vi "SRU2（DBL）.vi"(6 "复位":bool, 7 "启用（T）":bool=TRUE, 9 "初始值":dbl, 10 "Xi":dbl) -> (1 "Xi-1":dbl format="%.2f", 2 "Xi-2":dbl format="%.2f")   [LabVIEW 2012]
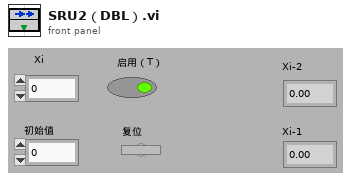
[diagram p1: front panel]
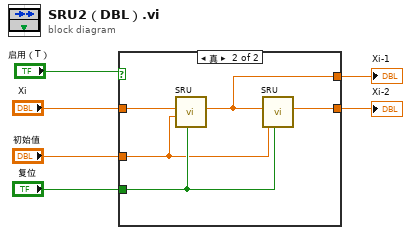
[diagram p0: block diagram]
diagram:
  n1 = case shown="真" "启用（T）" {
    tunnel: "复位" -> [_ w11]
    tunnel: "Xi" -> [w7 w10]
    tunnel: [w7 w12] -> w4
    tunnel: "初始值" -> [_ w9]
    tunnel: [w7 w8] -> w1
    frame False {
    }
    frame True {
      n2 = call-poly "SRU.vi"("复位"=w11, "初始值"=w9, "输入"=w10) -> ("上次值"=w8:dbl)  [unwired: 6 in, 2 out]
      n3 = call-poly "SRU.vi"("复位"=w11, "初始值"=w9, "输入"=w8) -> ("上次值"=w12:dbl)  [unwired: 6 in, 2 out]
    }
  }
  "Xi-2" <- w4
  "Xi-1" <- w1
